vi "PH_PPMA_PowerUnit.PC_StateRoss.vi"(0 "i ref in":refnum<vi>, 3 "Ross Status":T1 caption="Enabling State" items=["no info", "off/false/out", "on/true/in", "Failure", "Alarm", "Status 1", "Status 2", "Status 3"], 4 "not linked?":bool, 5 "error in (no error)":errorcluster) -> (14 "i ref out":refnum<vi>, 19 "error out":errorcluster)   [LabVIEW 2014, in "PH_PPMA_PowerUnit.lvlib"]
doc: "This VI writes the RR Tag values to own attributes, calculates the state of the device and sets the GUI object."
uses:
  PH_PPMA_PowerUnit.lvlib
  PH_StatusHandler/PH_StatusHandler.Status.ctl
  PH_Common/PH_Common.lvlib
  CSCore/BaseSM/BaseSM.lvlib
  PH_StatusHandler/PH_StatusHandler.lvlib
  PH_Beckhoff_PP_PU/PH_Beckhoff_PP_PU.lvlib
  PH_PowerUnit_BaseClass/PH_PowerUnit_BaseClass.lvlib
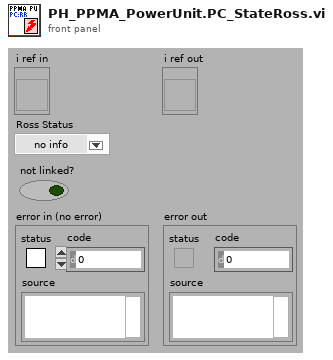
[diagram p1: front panel]
types:
  T1 = typedef "PH_StatusHandler.lvlib/PH_StatusHandler.Status.ctl" = i16
  T2 = typedef "PH_PPMA_PowerUnit.lvlib/PH_PPMA_PowerUnit.i attribute.ctl" = cluster{"GUI Refs":cluster{"Rods":refnum<vi>, "Ignitron":refnum<vi>, "Rossrelais":refnum<vi>, "Set Voltage":refnum<vi>, "PSU":refnum<vi>, "EOC":refnum<vi>, "Trigger":refnum<vi>}, "Rods":T3, "PSU":T4, "Ross Relais":T5, "Ignitron":T6, "Trigger":cluster{"State Device":T1, "linked?":bool}, "Timing Settings":cluster{"Prdc Fast?":bool, "Default Value Periodic Interval":i32, "Mercury on since":dbl, "Warm up Time Mercury [s]":dbl}, "Set Voltage [V]":dbl}
  T3 = typedef "PH_PPMA_PowerUnit.lvlib/PH_PPMA_PowerUnit.Rods Attributes.ctl" = cluster{"Instancename":string, "Device Status":T1, "linked?":bool}
  T4 = typedef "PH_PP_Common.lvlib/PH_PP_Common.PSU Attributes.ctl" = cluster{"lower limit [V]":dbl, "upper limit [V]":dbl, "Voltage set":bool, "State Device":T1, "linked?":bool}
  T5 = typedef "PH_PP_Common.lvlib/PH_PP_Common.Ross Relais Attributes.ctl" = cluster{"State Device":T1, "linked?":bool}
  T6 = typedef "PH_PP_Common.lvlib/PH_PP_Common.Ignitron Attributes.ctl" = cluster{"State Device":T1, "linked?":bool}
  T7 = typedef "PH_PowerUnit_BaseClass.lvlib/PH_PowerUnit_BaseClass.i attribute.ctl" = cluster{"Constructor finished":bool, "PU":cluster{"In use":bool, "Service ID in use":i32, "GUI Ref":refnum<vi>}, "Enabling":cluster{"State":T8, "GUI Ref":refnum<vi>}, "Timing":cluster{"Last Shot":dbl, "Time between Shots [Sec]":dbl, "Waiting Time over?":bool, "Service ID Waiting Time":i32, "GUI Ref":refnum<vi>, "Instance":cluster{"Status":T1, "linked?":bool, "GUI Ref":refnum<vi>}}, "Sequencer":cluster{"SM State":string, "GUI Ref":refnum<vi>, "linked":bool}, "Subscribed Trendmssgs":cluster{"Tagname":string, "Status":T1, "linked?":bool, "Shot Condition":T1, "GUI Ref":refnum<vi>}[], "PP PU":T9, "Default Voltage (V)":dbl, "GUI Refs":T10, "PSDB data":cluster{"Shot Voltage [V]":dbl, "State TO SM":T11, "Write 2 early":bool}, "State TO SM":T11}
  T8 = typedef "PH_SystemInformation.lvlib/PH_SystemInformationEnabling State.ctl" = i32
  T9 = typedef "PH_PP_Common.lvlib/PH_PP_Common.PUs.ctl" = enum16{"no Info", "PA-19mm-1", "PA-19mm-2", "PA-45mm-PILC", "PA-45mm-MAIN", "MA-PU-1", "MA-PU-2", "MA-PU-3", "MA-PU-4", "MA-PU-5", "MA-PU-6", "MA-FR", "MA-PILC", "PA-45mm-DP"}
  T10 = typedef "PH_PowerUnit_BaseClass.lvlib/PH_PowerUnit_BaseClass.GUI Refs.ctl" = cluster{"Delete Inst":refnum<vi>, "State TO SM":refnum<vi>, "State SM":refnum<vi>, "Fire":refnum<vi>}
  T11 = typedef "PH_PowerUnit_BaseClass.lvlib/PH_PowerUnit_BaseClass.SM States.ctl" = enum16{".", "Stand by", "Switch PU on", "Configure", "Set Default Voltage", "Set STANDBY", "Set READY", "Wait for Shot Cmd", "Open Dump Rods", "Open Ross Relais", "Close Ross Relais", "Switch PSU on", "Switch PSU off", "Charge", "Switch GD Channel on", "Close Dump Rods", "Rods-TO", "RR-TO", "PSU-TO", "Trigger-TO"}
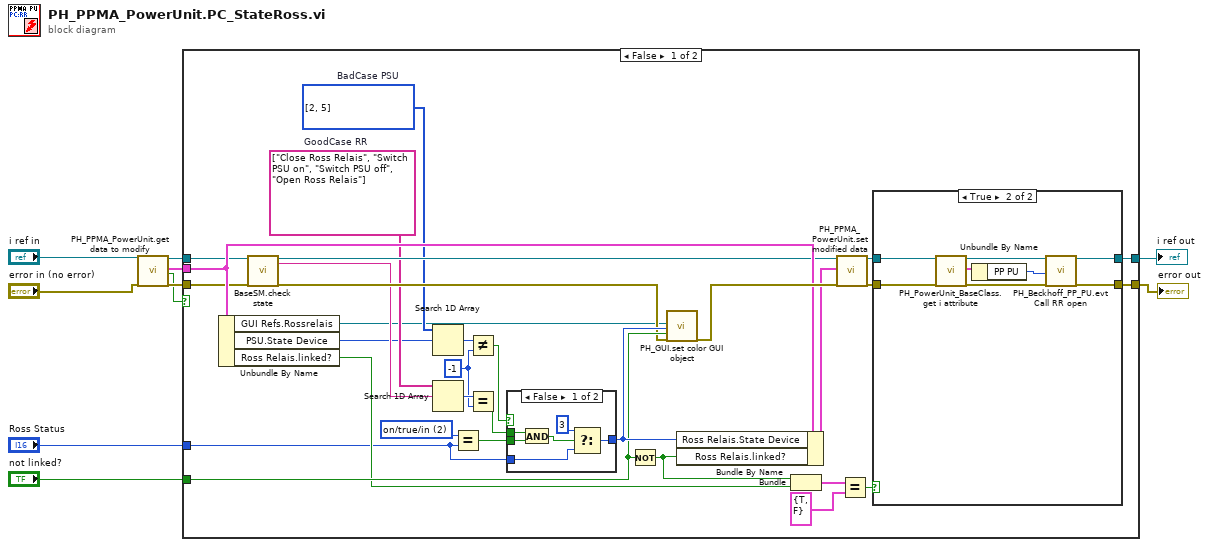
[diagram p0: block diagram]
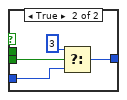
[diagram p2: hidden frame]
diagram:
  n1 = call "PH_PPMA_PowerUnit.get data to modify.vi"("i ref in"="i ref in", "error in (no error)"="error in (no error)") -> ("i ref out"=w10:refnum<vi>, "i attribute"=w8:T2, "timed out"=w7:bool, "error out"=w9:errorcluster)  [unwired: 14 in]
  n2 = case shown="False" w7 {
    tunnel: w10 -> [w28 w63]
    tunnel: [w35 w63] -> w4
    tunnel: w9 -> [w26 w62]
    tunnel: [w33 w62] -> w3
    tunnel: w8 -> [w38 _]
    tunnel: "Ross Status" -> [w23 _]
    tunnel: "not linked?" -> [w37 _]
    frame False {
      w17 = T1[] [2, 5] items=["no info", "off/false/out", "on/true/in", "Failure", "Alarm", "Status 1", "Status 2", "Status 3"]  # BadCase PSU
      w21 = string[] ["Close Ross Relais", "Switch PSU on", "Switch PSU off", "Open Ross Relais"]  # GoodCase RR
      w22 = T1 2 items=["no info", "off/false/out", "on/true/in", "Failure", "Alarm", "Status 1", "Status 2", "Status 3"] ("Ross Status")
      w16 = -1 ("index of element")
      n3 = Unbundle By Name(w38) -> ("GUI Refs.Rossrelais"=w11:refnum<vi>, "PSU.State Device"=w12:T1, "Ross Relais.linked?"=w32:bool)
      n4 = call "BaseSM.check state.vi"("i ref in"=w28, "error in (no error)"=w26) -> ("i ref out"=w27:refnum<vi>, "actualState"=w20:string, "error out"=w25:errorcluster)  [unwired: 12 in, 3 out]
      n5 = Search 1D Array(1D array=w17, element=w12) -> (index of element=w18:i32)  [unwired: 1 in]
      n6 = Search 1D Array(1D array=w21, element=w20) -> (index of element=w19:i32)  [unwired: 1 in]
      n7 = Equal?(x=w22, y=w23) -> (x = y?=w15:bool)
      n8 = Not Equal?(x=w18, y=w16) -> (x != y?=w14:bool)
      n9 = Equal?(x=w19, y=w16) -> (x = y?=w13:bool)
      n10 = case shown="False" w14 {
        tunnel: [w45 w51] -> w39
        tunnel: w23 -> [w46 w50]
        tunnel: w15 -> [w43 w48]
        tunnel: w13 -> [w44 _]
        frame False {
          n11 = And(x=w44, y=w43) -> (x .and. y?=w42:bool)
          n12 = Select(t=3, s=w42, f=w46) -> (s? t:f=w45:i32)
        }
        frame True {
          n13 = Select(t=3, s=w48, f=w50) -> (s? t:f=w51:i32)
        }
      }
      n14 = Not(x=w37) -> (.not. x?=w24:bool)
      n15 = call "PH_GUI.set color GUI object.vi"("GUI object Ref"=w11, "State"=w39, "Blinking? (false)"=w37, "error in (no error)"=w25) -> ("error out"=w41:errorcluster)  [unwired: 15 in]
      n16 = Bundle By Name(cluster=w38, "Ross Relais.State Device"=w39, "Ross Relais.linked?"=w24) -> (w40:T2)
      n17 = Bundle(w24, "linked?"=w32) -> (w31:cluster{bool, "linked?":bool})  [unwired: 1 in]
      n18 = call "PH_PPMA_PowerUnit.set modified data.vi"("i ref in"=w27, "i attribute"=w40, "error in (no error)"=w41) -> ("i ref out"=w36:refnum<vi>, "error out"=w34:errorcluster)  [unwired: 15 in]
      n19 = Equal?(x=w31, y=cluster{"linked?":bool, bool} {"linked?"=TRUE, FALSE}) -> (x = y?=w29:bool)
      n20 = case shown="True" w29 {
        tunnel: w36 -> [w52 w54]
        tunnel: [w52 w61] -> w35
        tunnel: w34 -> [w53 w55]
        tunnel: [w53 w60] -> w33
        frame False {
        }
        frame True {
          n21 = call "PH_PowerUnit_BaseClass.get i attribute.vi"("i ref in"=w54, "error in (no error)"=w55) -> ("i ref out"=w58:refnum<vi>, "i attribute"=w57:T7, "error out"=w59:errorcluster)  [unwired: 15 in]
          n22 = Unbundle By Name(w57) -> ("PP PU"=w56:T9)
          n23 = call "PH_Beckhoff_PP_PU.evt Call RR open.vi"("i ref in"=w58, "PU"=w56, "error in"=w59) -> ("i ref out"=w61:refnum<vi>, "error out"=w60:errorcluster)  [unwired: 15 in]
        }
      }
    }
    frame True {
    }
  }
  "error out" <- w3
  "i ref out" <- w4
